vi "RS232通訊-Write.vi"(8 "error in (no error)":errorcluster, 10 "string":string, 11 "VISA Refnum in":refnum<visa-resource-name>) -> (0 "error out":errorcluster, 2 "read buffer":string, 3 "VISA resource name out":refnum<visa-resource-name>)   [LabVIEW 2013]
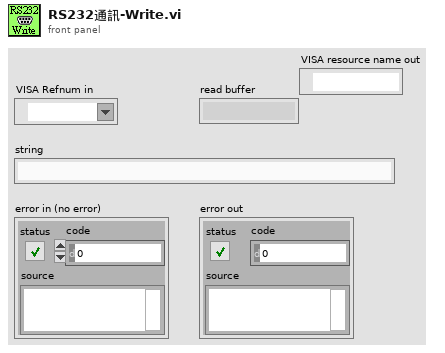
[diagram p1: front panel]
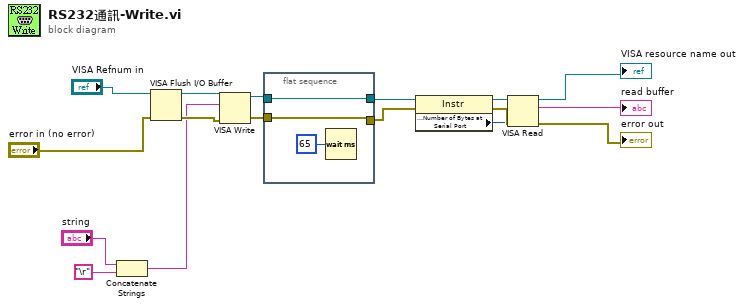
[diagram p0: block diagram]
diagram:
  n1 = Concatenate Strings("string", "\r") -> (w1:string)
  n2 = VISA Flush I/O Buffer(VISA resource name="VISA Refnum in", error in (no error)="error in (no error)") -> (VISA resource name out=w4:refnum<visa-resource-name>, error out=w2:errorcluster)  [unwired: 1 in]
  n3 = VISA Write(VISA resource name=w4, write buffer=w1, error in (no error)=w2) -> (VISA resource name out=w12:refnum<visa-resource-name>, error out=w13:errorcluster)  [unwired: 1 out]
  n4 = flat-sequence {
    tunnel: [w20] -> w8
    tunnel: w12 -> [w20]
    tunnel: [w19] -> w9
    tunnel: w13 -> [w19]
    frame #0 {
      n5 = Wait (ms)(milliseconds to wait=u32 65) -> ()  [unwired: 1 out]
    }
  }
  n6 = property class="Instr"(reference=w8, error in=w9) -> (reference out=w7:refnum<visa-resource-name>, error out=w10:errorcluster, "Serial Settings:Number of Bytes at Serial Port"=w6:u32)
  n7 = VISA Read(VISA resource name=w7, byte count=w6, error in (no error)=w10) -> (VISA resource name out=→"VISA resource name out":refnum<visa-resource-name>, read buffer=→"read buffer":string, error out=→"error out":errorcluster)  [unwired: 1 out]
